vi "Teleop.vi"(10 "Match Info":T1={"Autonomous Elapsed Seconds"=0.0, "TeleOp Elapsed Seconds"=0.0, "Disabled Elapsed Seconds"=0.0, "Visited Autonomous"=FALSE, "Visited TeleOp"=FALSE, "Visited Disabled"=FALSE, "Autonomous Settings"={"Autonomous Style"=enum."Independent", "VI Refnum"=refnum}}, 11 "Call Context":T2) -> ()   [LabVIEW 2011]
doc: "This VI is called for each TeleOp packet received from the DS where the robot is not disabled. It is often used to read from the joysticks and update I/O or to update setpoints for timed control loops. It should complete and return within 20 milliseconds or it may miss DS packets."
uses:
  <vilib>/Rock Robotics/WPI/DriverStation/WPI_DriverStationDerivedRobotMode.ctl
  <vilib>/Rock Robotics/WPI/DriverStation/WPI_DriverStationMatch Info.ctl
  Shared/Shooter Control Mode.ctl
  Robot Global Data.vi
  Shooter Global.vi
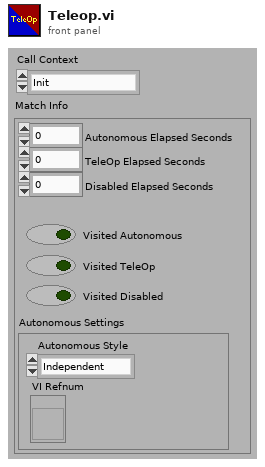
[diagram p1: front panel]
types:
  T1 = typedef "WPI_DriverStationMatch Info.ctl" = cluster{"Autonomous Elapsed Seconds":dbl, "TeleOp Elapsed Seconds":dbl, "Disabled Elapsed Seconds":dbl, "Visited Autonomous":bool, "Visited TeleOp":bool, "Visited Disabled":bool, "Autonomous Settings":cluster{"Autonomous Style":enum16{"Iterative", "Independent"}, "VI Refnum":refnum<vi>}}
  T2 = typedef "WPI_DriverStationDerivedRobotMode.ctl" = enum16{"Init", "Execute", "Stop"}
  T3 = cluster{"Analog 1":dbl, "Analog 2":dbl, "Analog 3":dbl, "Analog 4":dbl, "Analog 5":dbl, "Analog 6":dbl, "Analog 7":dbl, "Analog 8":dbl}
  T4 = typedef "WPI_JoystickDevRef.ctl" = cluster{"Device":T5}
  T5 = typedef "WPI_JoystickDeviceEnum.ctl" = enum16{"USB 1", "USB 2", "USB 3", "USB 4", "Kinect 1", "Kinect 2"}
  T6 = cluster{"axis 1 (x)":dbl, "axis 2 (y)":dbl, "axis 3 (throttle)":dbl, "axis 4":dbl, "axis 5":dbl, "axis 6":dbl}
  T7 = typedef "WPI_JoystickButtonState.ctl" = cluster{"Button 1":bool, "Button 2":bool, "Button 3":bool, "Button 4":bool, "Button 5":bool, "Button 6":bool, "Button 7":bool, "Button 8":bool, "Button 9":bool, "Button 10":bool, "Button 11":bool, "Button 12":bool}
  T8 = typedef "Drive Base Dashboard Package.ctl" = cluster{"Left":dbl, "Right":dbl, "Shifter":T9}
  T9 = typedef "Shifter State.ctl" = enum16{"Unknown", "Low", "High"}
  T10 = typedef "WPI_RobotDriveDevRef.ctl" = cluster{"DevStatus":errorcluster, "Motors[]":T11[], "Square Inputs":bool, "Max Output":dbl, "Isochronous":bool}
  T11 = typedef "WPI_MotorControlDeviceRef.ctl" = cluster{"DeviceStatus":errorcluster, "Type":enum16{"PWM", "CAN"}, "PWM":cluster{"Digital Module":T12, "PWM Channel":T13, "DeadBand":T14}, "CAN":cluster{"Device Number":u8, "Control Mode":T15, "Semaphore":T16, "Max Vout":dbl}, "Invert":bool, "TransformRef":T17, "InvTransformRef":T17}
  T12 = typedef "FPGA_TypedefDigitalModule.ctl" = enum16{"Digital Module 1", "Digital Module 2"}
  T13 = typedef "FPGA_DIOPWMChannel.ctl" = enum8{"PWM 1", "PWM 2", "PWM 3", "PWM 4", "PWM 5", "PWM 6", "PWM 7", "PWM 8", "PWM 9", "PWM 10", "Invalid"}
  T14 = typedef "WPI_PWMDeadband.ctl" = cluster{"Name":string, "maxPositivePwm":i32, "minPositivePwm":i32, "centerPwm":i32, "maxNegativePwm":i32, "minNegativePwm":i32, "angularRange":u16}
  T15 = typedef "WPI_CANJaguar_ControlMode.ctl" = enum8{"Percent VBus", "Current", "Speed", "Position", "Voltage"}
  T16 = typedef "Semaphore RefNum" = refnum<k1>
  T17 = typedef "WPI_PWMTransform_ConPane.ctl" = refnum<vi>
  T18 = typedef "Shooter Control Mode.ctl" = enum16{"Key", "Mid Field", "Backfield", "Topspin", "Open Loop Control", "Off"}
  T19 = enum16{"Off", "Open Loop Control", "Closed Loop Control", "Top Spin"}
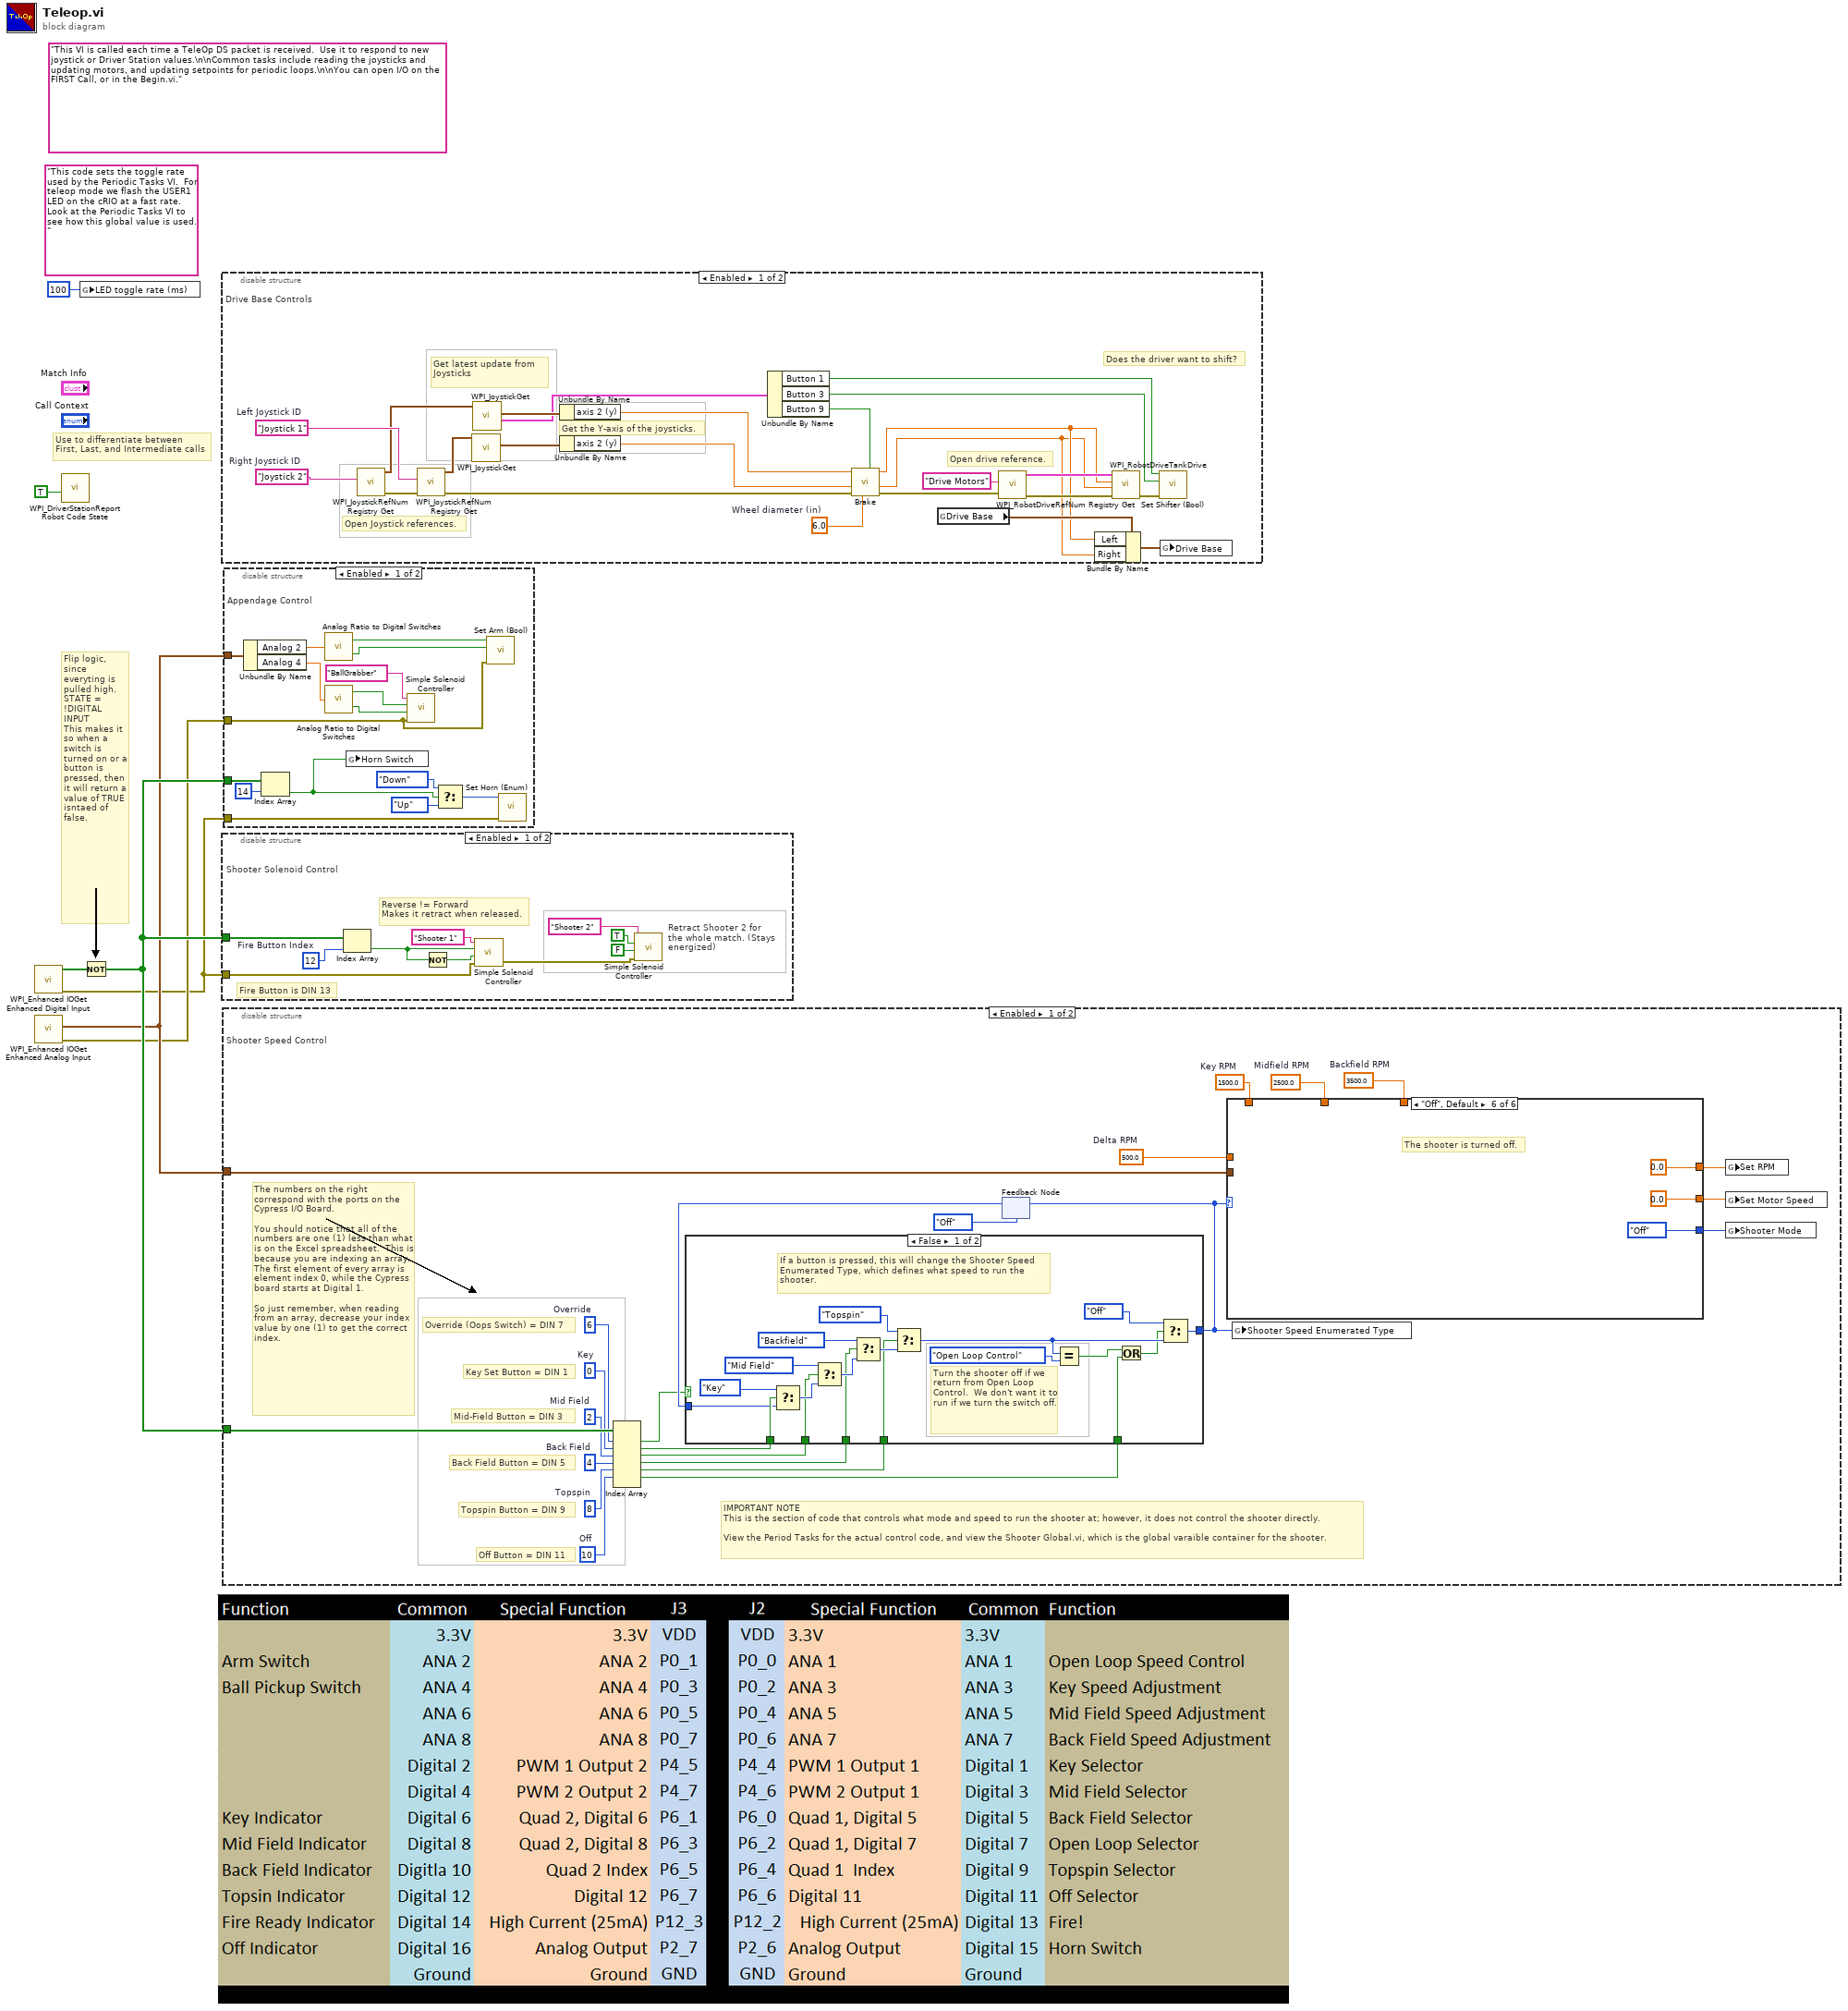
[diagram p0: block diagram]
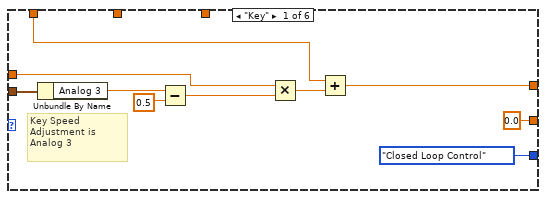
[diagram p2: hidden frame]
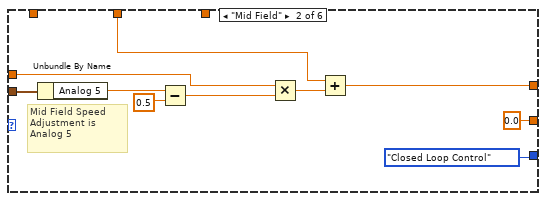
[diagram p3: hidden frame]
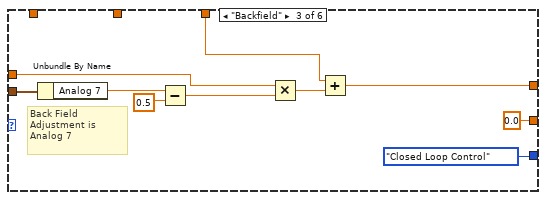
[diagram p4: hidden frame]
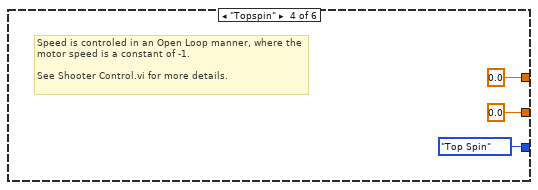
[diagram p5: hidden frame]
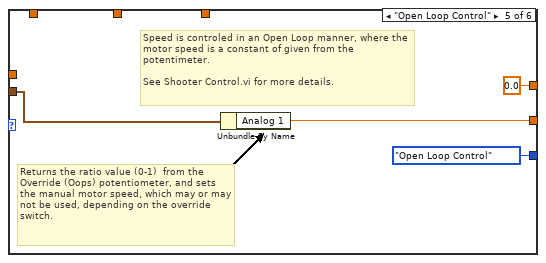
[diagram p6: hidden frame]
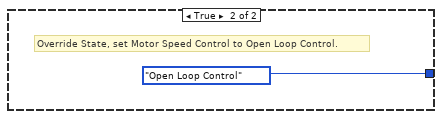
[diagram p7: hidden frame]
diagram:
  (unwired) "This code sets the toggle rate used by the Periodic Tasks VI.  For teleop mode we flash the USER1 LED on the cRIO at a fast rate.  Look at the Periodic Tasks VI to see how this global value is used."
  (unwired) "This VI is called each time a TeleOp DS packet is received.  Use it to respond to new joystick or Driver Station values.\n\nCommon tasks include reading the joysticks and updating motors, and updating setpoints for periodic loops.\n\nYou can open I/O on the FIRST Call, or in the Begin.vi."
  # "Flip logic, since everyting is pulled high.\nSTATE = !DIGITAL INPUT\nThis makes it so when a switch is turned on or a button is pressed, then it will return a value of TRUE isntaed of false."
  # "Use to differentiate between\nFirst, Last, and Intermediate calls"
  n1 = call <vilib>:"WPI_Enhanced IOGet Enhanced Digital Input.vi"() -> ("error out"=w1:errorcluster, "Digital Input [1-16]"=w5:bool[])  [unwired: 10 in]
  n2 = call <vilib>:"WPI_Enhanced IOGet Enhanced Analog Input.vi"() -> ("error out"=w2:errorcluster, "Analog Ratios (0-1)"=w3:T3)  [unwired: 9 in, 1 out]
  n3 = call <vilib>:"WPI_DriverStationReport Robot Code State.vi"("TeleOp"=TRUE ("Autonomous")) -> ()  [unwired: 10 in, 1 out]
  n4 = global write "Robot Global Data.vi" "LED toggle rate (ms)"(u32 100 ("LED ms toggle rate")) -> ()
  n5 = Not(x=w5) -> (.not. x?=w4:bool[])
  n6 = disable-structure shown="Enabled" {
    frame Enabled {
      w13 = 6.0  # Wheel diameter (in)
      w27 = "Joystick 2"  # Right Joystick ID
      w29 = "Joystick 1"  # Left Joystick ID
      # "Get latest update from Joysticks"
      # "Does the driver want to shift?"
      # "Get the Y-axis of the joysticks."
      # "Open drive reference."
      # "Open Joystick references."
      # "Drive Base Controls"
      n7 = call <vilib>:"WPI_JoystickRefNum Registry Get.vi"("refnum name"=w27) -> ("error out"=w25:errorcluster, "JoystickDevRef"=w26:T4)  [unwired: 1 in, 8 out]
      n8 = call <vilib>:"WPI_JoystickRefNum Registry Get.vi"("error in (no error)"=w25, "refnum name"=w29) -> ("error out"=w15:errorcluster, "JoystickDevRef"=w28:T4)  [unwired: 8 out]
      n9 = call <vilib>:"WPI_JoystickGet.vi"("JoystickDevRef"=w28) -> ("Axes"=w30:T6)  [unwired: 1 in, 5 out]
      n10 = call <vilib>:"WPI_JoystickGet.vi"("JoystickDevRef"=w26) -> ("Buttons"=w23:T7, "Axes"=w24:T6)  [unwired: 1 in, 4 out]
      n11 = Unbundle By Name(w24) -> ("axis 2 (y)"=w16:dbl)
      n12 = Unbundle By Name(w30) -> ("axis 2 (y)"=w17:dbl)
      n13 = Unbundle By Name(w23) -> ("Button 1"=w20:bool, "Button 3"=w19:bool, "Button 9"=w12:bool)
      n14 = call "Brake.vi"("Brake?"=w12, "Wheel diameter (in)"=w13, "error in (no error)"=w15, "Right Speed"=w17, "Left Speed"=w16) -> ("error out"=w14:errorcluster, "Right Output"=w8:dbl, "Left Output"=w9:dbl)  [unwired: 2 in]
      n15 = global read "Robot Global Data.vi" "Drive Base"() -> (w11:T8)
      n16 = call <vilib>:"WPI_RobotDriveRefNum Registry Get.vi"("error in (no error)"=w14, "refnum name"="Drive Motors") -> ("error out"=w21:errorcluster, "RobotDriveDevRef"=w22:T10)  [unwired: 8 out]
      n17 = Bundle By Name(cluster=w11, "Left"=w9, "Right"=w8) -> (w10:T8)
      n18 = call <vilib>:"WPI_RobotDriveTankDrive.vi"("error in (no error)"=w21, "Right axis value"=w8, "Left axis value"=w9, "RobotDriveDevRef"=w22) -> ("error out"=w18:errorcluster)  [unwired: 6 in, 1 out]
      n19 = call "Set Shifter (Bool).vi"("error in (no error)"=w18, "Low"=w19, "High"=w20) -> ()  [unwired: 8 in, 1 out]
      n20 = global write "Robot Global Data.vi" "Drive Base"(w10) -> ()
    }
    frame Disabled {
    }
  }
  n21 = disable-structure shown="Enabled" {
    disable-tunnel: w4 -> [w41 _]
    disable-tunnel: w1 -> [w32 _]
    frame Enabled {
      w38 = 12  # Fire Button Index
      # "Fire Button is DIN 13"
      # "Reverse != Forward\nMakes it retract when released."
      # "Retract Shooter 2 for the whole match. (Stays energized)"
      # "Shooter Solenoid Control"
      n22 = Index Array(array=w41, index=w38) -> (element=w36:bool)
      n23 = Not(x=w36) -> (.not. x?=w35:bool)
      n24 = call "Simple Solenoid Controller.vi"("error in (no error)"=w32, "Reverse"=w35, "Forward"=w36, "refnum name"="Shooter 1") -> ("error out"=w33:errorcluster)  [unwired: 6 in, 1 out]
      n25 = call "Simple Solenoid Controller.vi"("error in (no error)"=w33, "Reverse"=FALSE, "Forward"=TRUE, "refnum name"="Shooter 2") -> ()  [unwired: 6 in, 2 out]
    }
    frame Disabled {
    }
  }
  n26 = disable-structure shown="Enabled" {
    disable-tunnel: w4 -> [w65 _]
    disable-tunnel: w3 -> [w64 _]
    frame Enabled {
      w47 = 1500.0  # Key RPM
      w48 = 3500.0  # Backfield RPM
      w49 = 2500.0  # Midfield RPM
      w50 = 500.0  # Delta RPM
      w53 = 6  # Override
      w59 = 10  # Off
      w60 = 8  # Topspin
      w61 = 4  # Back Field
      w62 = 2  # Mid Field
      w63 = 0  # Key
      # "IMPORTANT NOTE\nThis is the section of code that controls what mode and speed to run the shooter at; however, it does not control the shooter directly.\n\nView the Period Tasks for the actual control code, and view the Shooter Global.vi, which is the global varaible container for the shooter."
      # "The numbers on the right correspond with the ports on the Cypress I/O Board.\n\nYou should notice that all of the numbers are one (1) less than what is on the Excel spreadsheet.  This is because you are indexing an array.  The first element of every array is element index 0, while the Cypress board starts at Digital 1.\n\nSo just remember, when reading from an array, decrease your index value by one (1) to get the correct index."
      # "Off Button = DIN 11"
      # "Topspin Button = DIN 9"
      # "Back Field Button = DIN 5"
      # "Mid-Field Button = DIN 3"
      # "Key Set Button = DIN 1"
      # "Override (Oops Switch) = DIN 7"
      # "Shooter Speed Control"
      n27 = Index Array(array=w65, index #1=w53, index #2=w63, index #3=w62, index #4=w61, index #5=w60, index #6=w59) -> (element #1=w52:bool, element #2=w57:bool, element #3=w56:bool, element #4=w55:bool, element #5=w54:bool, element #6=w43:bool)  [unwired: 1 in, 1 out]
      n28 = feedback #1(Shooter_Control_Mode."Off") -> (w58:T18)
      n29 = case shown="False" w52 {
        tunnel: w58 -> [w111 _]
        tunnel: [w112 Shooter_Control_Mode."Open Loop Control"] -> w44
        tunnel: w57 -> [w120 _]
        tunnel: w56 -> [w119 _]
        tunnel: w55 -> [w118 _]
        tunnel: w54 -> [w117 _]
        tunnel: w43 -> [w107 _]
        frame False {
          # "Turn the shooter off if we return from Open Loop Control.  We don't want it to run if we turn the switch off."
          # "If a button is pressed, this will change the Shooter Speed Enumerated Type, which defines what speed to run the shooter."
          n30 = Select(t=Shooter_Control_Mode."Key", s=w120, f=w111) -> (s? t:f=w123:T18)
          n31 = Select(t=Shooter_Control_Mode."Mid Field", s=w119, f=w123) -> (s? t:f=w122:T18)
          n32 = Select(t=Shooter_Control_Mode."Backfield", s=w118, f=w122) -> (s? t:f=w121:T18)
          n33 = Select(t=Shooter_Control_Mode."Topspin", s=w117, f=w121) -> (s? t:f=w110:T18)
          n34 = Equal?(x=w110, y=Shooter_Control_Mode."Open Loop Control") -> (x = y?=w108:bool)
          n35 = Or(x=w108, y=w107) -> (x .or. y?=w106:bool)
          n36 = Select(t=Shooter_Control_Mode."Off", s=w106, f=w110) -> (s? t:f=w112:T18)
        }
        frame True {
          # "Override State, set Motor Speed Control to Open Loop Control."
        }
      }
      n37 = feedback-in #1(w44) -> ()
      n38 = case shown="\"Off\", Default" w44 {
        tunnel: [w70 w82 w92 0.0 0.0 0.0] -> w51
        tunnel: w64 -> [w74 w80 w90 _ w99 _]
        tunnel: w50 -> [w72 w81 w91 _ _ _]
        tunnel: w49 -> [_ w78 _ _ _ _]
        tunnel: w48 -> [_ _ w89 _ _ _]
        tunnel: w47 -> [w68 _ _ _ _ _]
        tunnel: [T19."Closed Loop Control" ("Shooter Mode") T19."Closed Loop Control" ("Shooter Mode") T19."Closed Loop Control" ("Shooter Mode") T19."Top Spin" ("Shooter Mode") T19."Open Loop Control" ("Shooter Mode") T19."Off" ("Shooter Mode")] -> w46
        tunnel: [0.0 ("Analog 1") 0.0 ("Analog 1") 0.0 ("Analog 1") 0.0 ("Analog 1") w100 0.0 ("Analog 1")] -> w42
        frame "Key" {
          # "Key Speed Adjustment is Analog 3"
          n39 = Unbundle By Name(w74) -> ("Analog 3"=w71:dbl)
          n40 = Subtract(x=w71, y=0.5) -> (x-y=w69:dbl)
          n41 = Multiply(x=w72, y=w69) -> (x*y=w73:dbl)
          n42 = Add(x=w68, y=w73) -> (x+y=w70:dbl)
        }
        frame "Mid Field" {
          # "Mid Field Speed Adjustment is Analog 5"
          n43 = Unbundle By Name(w80) -> ("Analog 5"=w83:dbl)
          n44 = Subtract(x=w83, y=0.5) -> (x-y=w79:dbl)
          n45 = Multiply(x=w81, y=w79) -> (x*y=w84:dbl)
          n46 = Add(x=w78, y=w84) -> (x+y=w82:dbl)
        }
        frame "Backfield" {
          # "Back Field Adjustment is Analog 7"
          n47 = Unbundle By Name(w90) -> ("Analog 7"=w93:dbl)
          n48 = Subtract(x=w93, y=0.5) -> (x-y=w88:dbl)
          n49 = Multiply(x=w91, y=w88) -> (x*y=w94:dbl)
          n50 = Add(x=w89, y=w94) -> (x+y=w92:dbl)
        }
        frame "Topspin" {
          # "Speed is controled in an Open Loop manner, where the motor speed is a constant of -1.\n\nSee Shooter Control.vi for more details."
        }
        frame "Open Loop Control" {
          # "Returns the ratio value (0-1)  from the Override (Oops) potentiometer, and sets the manual motor speed, which may or may not be used, depending on the override switch."
          # "Speed is controled in an Open Loop manner, where the motor speed is a constant of given from the potentimeter.\n\nSee Shooter Control.vi for more details."
          n51 = Unbundle By Name(w99) -> ("Analog 1"=w100:dbl)
        }
        frame "Off", Default {
          # "The shooter is turned off."
        }
      }
      n52 = global write "Shooter Global.vi" "Shooter Speed Enumerated Type"(w44) -> ()
      n53 = global write "Shooter Global.vi" "Set RPM"(w51) -> ()
      n54 = global write "Shooter Global.vi" "Set Motor Speed"(w42) -> ()
      n55 = global write "Shooter Global.vi" "Shooter Mode"(w46) -> ()
    }
    frame Disabled {
    }
  }
  n56 = disable-structure shown="Enabled" {
    disable-tunnel: w4 -> [w141 _]
    disable-tunnel: w3 -> [w140 _]
    disable-tunnel: w1 -> [w139 _]
    disable-tunnel: w2 -> [w138 _]
    frame Enabled {
      # "Appendage Control"
      n57 = Unbundle By Name(w140) -> ("Analog 2"=w137:dbl, "Analog 4"=w136:dbl)
      n58 = Index Array(array=w141, index=14) -> (element=w127:bool)
      n59 = call "Analog Ratio to Digital Switches.vi"("Analog Ratio Input"=w137) -> ("High Output"=w131:bool, "Low Output"=w130:bool)
      n60 = call "Analog Ratio to Digital Switches.vi"("Analog Ratio Input"=w136) -> ("High Output"=w135:bool, "Low Output"=w134:bool)
      n61 = global write "Robot Global Data.vi" "Horn Switch"(w127) -> ()
      n62 = call "Simple Solenoid Controller.vi"("error in (no error)"=w138, "Reverse"=w134, "Forward"=w135, "refnum name"="BallGrabber") -> ()  [unwired: 6 in, 2 out]
      n63 = Select(t=enum16{"Down", "Up"}."Down" ("Horn"), s=w127, f=enum16{"Down", "Up"}."Up") -> (s? t:f=w126:enum16{"Down", "Up"})
      n64 = call "Set Arm (Bool).vi"("error in (no error)"=w138, "Down"=w130, "Up"=w131) -> ()  [unwired: 8 in, 1 out]
      n65 = call "Set Horn (Enum).vi"("error in (no error)"=w139, "Horn"=w126) -> ()  [unwired: 9 in, 1 out]
    }
    frame Disabled {
    }
  }
